vi "Blocking.vi"(3 "Blocking requirements":cluster{"Value":dbl, " Number":i32}[](array[cluster])) -> (1 "Blocking array":dbl[](array[numeric]))   [LabVIEW 2013]
panel:
  in  "stop":bool
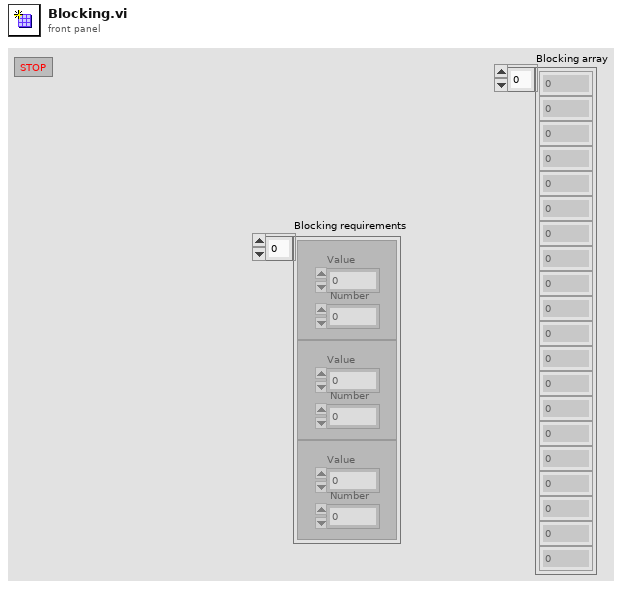
[diagram p1: front panel]
types:
  T1 = cluster{"number: 0 to 1":dbl, "number: 0 to 1":dbl}[]
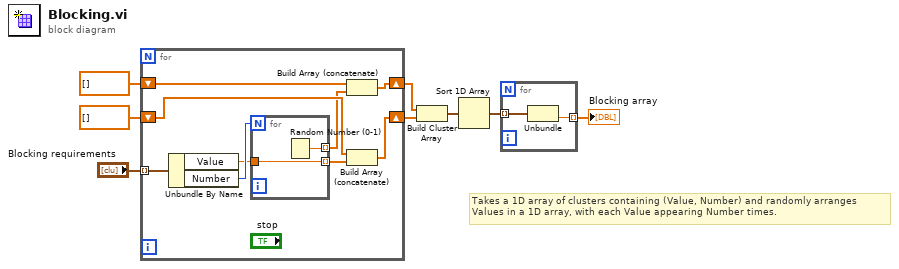
[diagram p0: block diagram]
diagram:
  # "Takes a 1D array of clusters containing (Value, Number) and randomly arranges\nValues in a 1D array, with each Value appearing Number times."
  n1 = for {
    tunnel: "Blocking requirements" -> [w17] mode=indexing
    shift-right: [w12] -> w1
    shift-left: dbl[] [] -> [w14]
    shift-right: [w10] -> w2
    shift-left: dbl[] [] -> [w9]
    n2 = Unbundle By Name(w17) -> ("Value"=w15:dbl, "Number"=w16:i32)
    n3 = for {
      N: w16 -> [_]
      tunnel: w15 -> [w19]
      tunnel: [w19] -> w13 mode=indexing
      tunnel: [w18] -> w11 mode=indexing
      n4 = Random Number (0-1)() -> (number: 0 to 1=w18:dbl)
    }
    n5 = Build Array (concatenate)(w9, w11) -> (w10:dbl[])
    n6 = Build Array (concatenate)(w14, w13) -> (w12:dbl[])
  }
  n7 = Build Cluster Array(w2, w1) -> (w5:T1)
  n8 = Sort 1D Array(array=w5) -> (sorted array=w7:T1)
  n9 = for {
    tunnel: w7 -> [w21] mode=indexing
    tunnel: [w20] -> w6 mode=indexing
    n10 = Unbundle(w21) -> ("number: 0 to 1"=w20:dbl)  [unwired: 1 out]
  }
  "Blocking array" <- w6
